vi "UsrProfiles-Remove unticked changes.vi"(0 "Changes array ctrl":refnum<vi>, 5 "Keys of changed parameters-DBL":T3, 7 "Keys of changed parameters-STRING":T1, 9 "Keys of changed parameters-BOOL":T5, 11 "error in (no error)":errorcluster) -> (4 "Some values to be saved":bool, 6 "Keys of changed parameters-DBL":T3, 8 "Keys of changed parameters-STRING":T1, 10 "Keys of changed parameters-BOOL":T5, 15 "error out":errorcluster)   [LabVIEW 2020]
uses:
  Typedefs/Changes info cluster-BOOL.ctl
  Configuration code/Typedefs/Ini file interface (Boolean).ctl
  Typedefs/Changes info cluster-DBL.ctl
  Configuration code/Typedefs/Ini file interface (DBL).ctl
  Typedefs/Changes info cluster-STRING.ctl
  Configuration code/Typedefs/Ini file interface (String).ctl
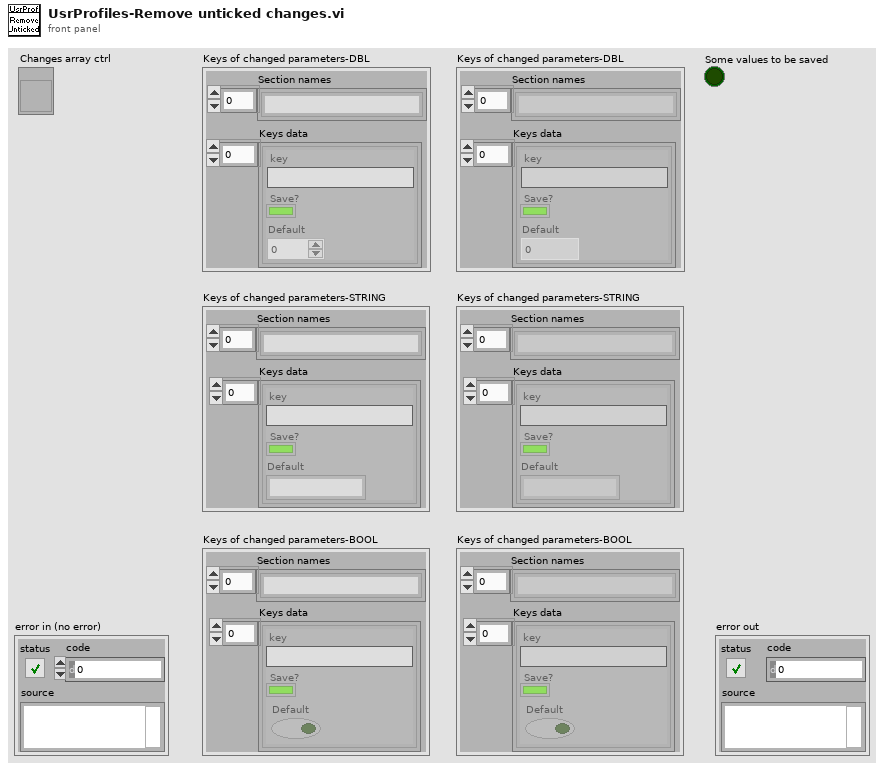
[diagram p1: front panel]
types:
  T1 = typedef "Changes info cluster-STRING.ctl" = cluster{"Section names":string[], "Keys data":T2}
  T2 = typedef "Ini file interface (String).ctl" = cluster{"key":string, "Save?":bool, "Default":string}[]
  T3 = typedef "Changes info cluster-DBL.ctl" = cluster{"Section names":string[], "Keys data":T4}
  T4 = typedef "Ini file interface (DBL).ctl" = cluster{"key":string, "Save?":bool, "Default":dbl}[]
  T5 = typedef "Changes info cluster-BOOL.ctl" = cluster{"Section names":string[], "Keys data":T6}
  T6 = typedef "Ini file interface (Boolean).ctl" = cluster{"key":string, "Save?":bool, "Default":bool}[]
  T7 = typedef "Changed parameter cluster.ctl" = cluster{"Name":string, "Old value":string, "New value":string, "Save":bool}
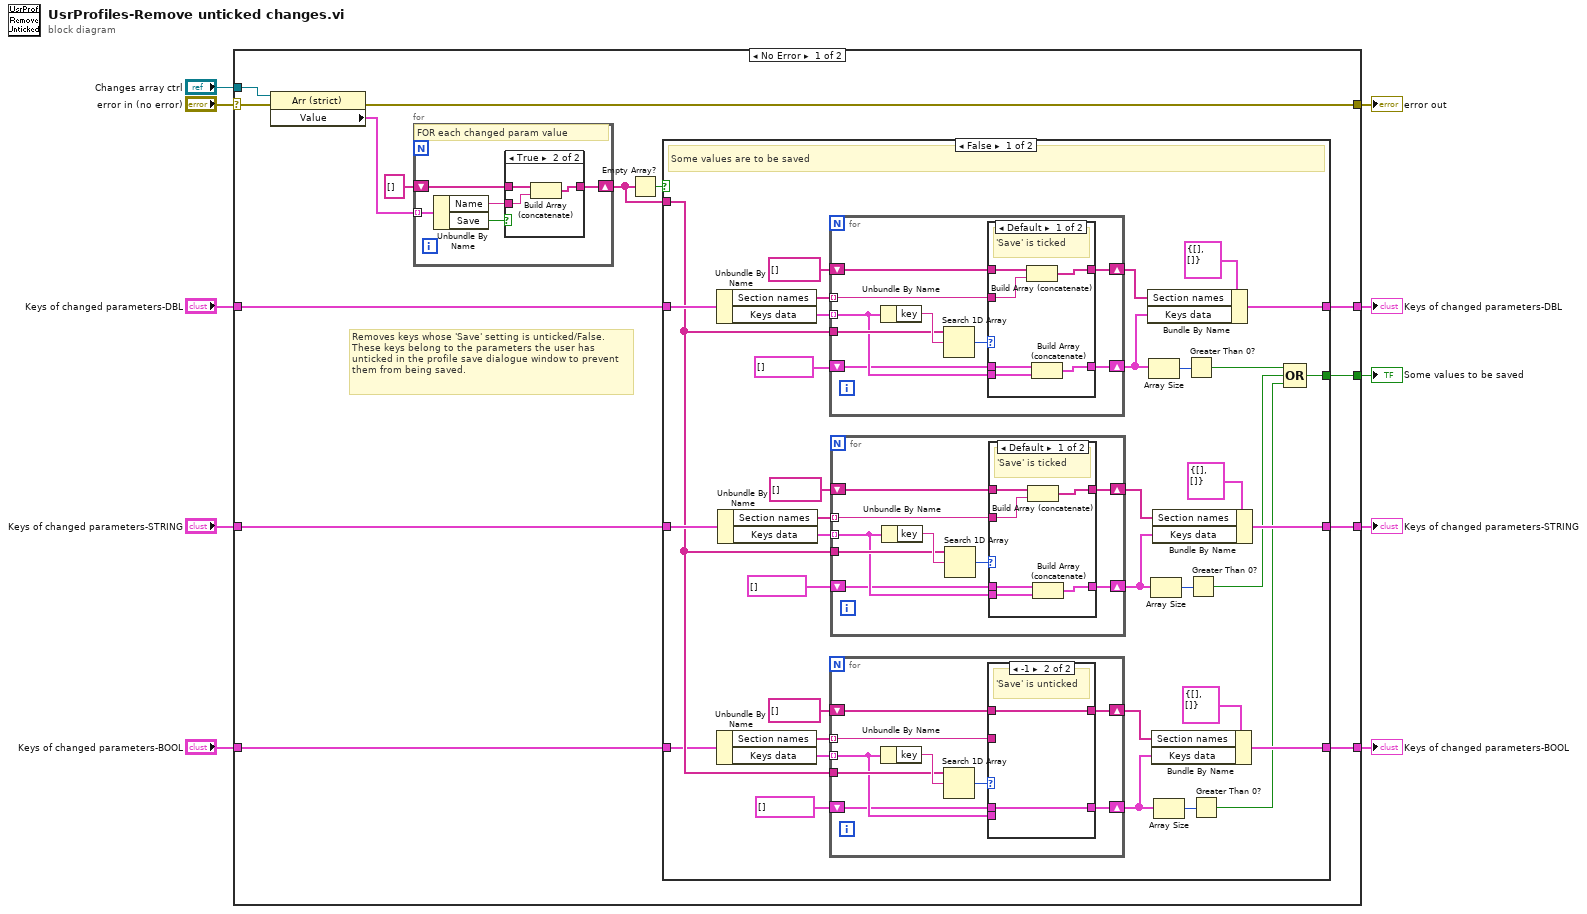
[diagram p0: block diagram]
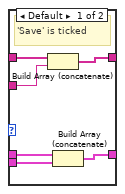
[diagram p2: hidden frame]
diagram:
  n1 = case shown="No Error" "error in (no error)" {
    selector: "error in (no error)" -> [w23 w120]
    tunnel: "Changes array ctrl" -> [w24 _]
    tunnel: [w22 w120] -> w8
    tunnel: "Keys of changed parameters-BOOL" -> [w12 _]
    tunnel: "Keys of changed parameters-DBL" -> [w17 _]
    tunnel: "Keys of changed parameters-STRING" -> [w16 _]
    tunnel: [w15 _] -> w4
    tunnel: [w14 _] -> w3
    tunnel: [w13 _] -> w2
    tunnel: [w11 _] -> w1
    frame No Error {
      # "Removes keys whose 'Save' setting is unticked/False.\nThese keys belong to the parameters the user has unticked in the profile save dialogue window to prevent them from being saved."
      n2 = property on="Property Node" class="Arr (strict)"(reference=w24, error in=w23) -> (error out=w22:errorcluster, "Value"=w21:T7[])  [unwired: 1 out]
      n3 = for {
        tunnel: w21 -> [w115] mode=indexing
        shift-right: [w112] -> w18
        shift-left: string[] [] -> [w111]
        # "FOR each changed param value"
        n4 = Unbundle By Name(w115) -> ("Name"=w113:string, "Save"=w114:bool)
        n5 = case shown="True" w114 {
          tunnel: w113 -> [_ w118]
          tunnel: [w116 w119] -> w112
          tunnel: w111 -> [w116 w117]
          frame False {
          }
          frame True {
            n6 = Build Array (concatenate)(w117, w118) -> (w119:string[])
          }
        }
      }
      n7 = Empty Array?(array=w18) -> (empty?=w19:bool)
      n8 = case shown="False" w19 {
        tunnel: w18 -> [w38 _]
        tunnel: w17 -> [w56 _]
        tunnel: w16 -> [w47 _]
        tunnel: [w57 _] -> w15
        tunnel: [w45 _] -> w14
        tunnel: [w36 _] -> w13
        tunnel: w12 -> [w37 _]
        tunnel: [w25 _] -> w11
        frame False {
          # "Some values are to be saved"
          n9 = Unbundle By Name(w56) -> ("Section names"=w55:string[], "Keys data"=w59:T4)
          n10 = Unbundle By Name(w37) -> ("Section names"=w42:string[], "Keys data"=w43:T6)
          n11 = Unbundle By Name(w47) -> ("Section names"=w50:string[], "Keys data"=w49:T2)
          n12 = for {
            tunnel: w59 -> [w99] mode=indexing
            tunnel: w38 -> [w100]
            shift-right: [w98] -> w34
            shift-left: T4 [] ("Keys data") -> [w97]
            tunnel: w55 -> [w96] mode=indexing
            shift-right: [w95] -> w53
            shift-left: string[] [] -> [w94]
            n13 = Unbundle By Name(w99) -> ("key"=w102:string)
            n14 = Search 1D Array(1D array=w100, element=w102) -> (index of element=w101:i32)  [unwired: 1 in]
            n15 = case shown="Default" w101 {
              tunnel: w99 -> [w108 _]
              tunnel: [w107 w110] -> w98
              tunnel: w97 -> [w106 w110]
              tunnel: w96 -> [w104 _]
              tunnel: [w105 w109] -> w95
              tunnel: w94 -> [w103 w109]
              frame Default {
                # "'Save' is ticked"
                n16 = Build Array (concatenate)(w103, w104) -> (w105:string[])
                n17 = Build Array (concatenate)(w106, w108) -> (w107:T4)
              }
              frame -1 {
                # "'Save' is unticked"
              }
            }
          }
          n18 = for {
            tunnel: w43 -> [w65] mode=indexing
            tunnel: w38 -> [w66]
            shift-right: [w64] -> w29
            shift-left: T6 [] ("Keys data") -> [w63]
            tunnel: w42 -> [w62] mode=indexing
            shift-right: [w61] -> w40
            shift-left: string[] [] -> [w60]
            n19 = Unbundle By Name(w65) -> ("key"=w68:string)
            n20 = Search 1D Array(1D array=w66, element=w68) -> (index of element=w67:i32)  [unwired: 1 in]
            n21 = case shown="-1" w67 {
              tunnel: w65 -> [w74 _]
              tunnel: [w73 w76] -> w64
              tunnel: w63 -> [w72 w76]
              tunnel: w62 -> [w70 _]
              tunnel: [w71 w75] -> w61
              tunnel: w60 -> [w69 w75]
              frame Default {
                # "'Save' is ticked"
                n22 = Build Array (concatenate)(w69, w70) -> (w71:string[])
                n23 = Build Array (concatenate)(w72, w74) -> (w73:T6)
              }
              frame -1 {
                # "'Save' is unticked"
              }
            }
          }
          n24 = for {
            tunnel: w49 -> [w82] mode=indexing
            tunnel: w38 -> [w83]
            shift-right: [w81] -> w31
            shift-left: T2 [] ("Keys data") -> [w80]
            tunnel: w50 -> [w79] mode=indexing
            shift-right: [w78] -> w52
            shift-left: string[] [] -> [w77]
            n25 = Unbundle By Name(w82) -> ("key"=w85:string)
            n26 = Search 1D Array(1D array=w83, element=w85) -> (index of element=w84:i32)  [unwired: 1 in]
            n27 = case shown="Default" w84 {
              tunnel: w82 -> [w91 _]
              tunnel: [w90 w93] -> w81
              tunnel: w80 -> [w89 w93]
              tunnel: w79 -> [w87 _]
              tunnel: [w88 w92] -> w78
              tunnel: w77 -> [w86 w92]
              frame Default {
                # "'Save' is ticked"
                n28 = Build Array (concatenate)(w86, w87) -> (w88:string[])
                n29 = Build Array (concatenate)(w89, w91) -> (w90:T2)
              }
              frame -1 {
                # "'Save' is unticked"
              }
            }
          }
          n30 = Bundle By Name(cluster=T3 {"Section names"=[], "Keys data"=[]} ("Keys of changed parameters-DBL"), "Section names"=w53, "Keys data"=w34) -> (w57:T3)
          n31 = Array Size(array=w34) -> (size(s)=w33:i32)
          n32 = Array Size(array=w31) -> (size(s)=w32:i32)
          n33 = Bundle By Name(cluster=T5 {"Section names"=[], "Keys data"=[]} ("Keys of changed parameters-BOOL"), "Section names"=w40, "Keys data"=w29) -> (w36:T5)
          n34 = Bundle By Name(cluster=T1 {"Section names"=[], "Keys data"=[]} ("Keys of changed parameters-STRING"), "Section names"=w52, "Keys data"=w31) -> (w45:T1)
          n35 = Array Size(array=w29) -> (size(s)=w30:i32)
          n36 = Greater Than 0?(x=w33) -> (x > 0?=w28:bool)
          n37 = Greater Than 0?(x=w32) -> (x > 0?=w27:bool)
          n38 = Greater Than 0?(x=w30) -> (x > 0?=w26:bool)
          n39 = Compound Arithmetic op=OR(w28, w27, w26) -> (w25:bool)
        }
        frame True {
          # "No values are to be saved"
        }
      }
    }
    frame Error {
    }
  }
  "error out" <- w8
  "Keys of changed parameters-BOOL" <- w2
  "Keys of changed parameters-DBL" <- w4
  "Keys of changed parameters-STRING" <- w3
  "Some values to be saved" <- w1
